vi "Fetch PRACH EVM Vs Subcarrier Trace Results.vi"(8 "error in (no error)":errorcluster, 9 "Result Type (Current)":i32(ring) items=["Current"=0, "Average"=1, "Maximum"=4], 10 "Instance (1)":T1=1, 11 "VISA resource name":refnum<visa-resource-name>) -> (0 "error out":errorcluster, 1 "Results":dbl[](array[numeric]) format="%^.3e", 2 "Reliability":i32, 3 "VISA resource name out":refnum<visa-resource-name>)   [LabVIEW 2020, in "Rohde&Schwarz CMWXP NR FR1 Measurement.lvlib"]
doc: "Returns the values of the EVM vs subcarrier traces. Each value is averaged over the samples in one preamble subcarrier.\n\nAttributes:\nRSCMWXPNRFR1M_ATTR_FETCH_PRACH_EVM_VS_SUBCARRIER_CURRENT_TRACE_RESULTS\nRSCMWXPNRFR1M_ATTR_FETCH_PRACH_EVM_VS_SUBCARRIER_AVERAGE_TRACE_RESULTS\nRSCMWXPNRFR1M_ATTR_FETCH_PRACH_EVM_VS_SUBCARRIER_MAXIMUM_TRACE_RESULTS\n\nRemote-control commands:\nFETCh:NRSub:MEAS<i>:PRACh:TRACe:EVM:CURRent?\nFETCh:NRSub:MEAS<i>:PRACh:TRACe:EVM:AVERage?\nFETCh:NRSub:MEAS<i>:PRACh:TRACe:EVM:MAXimum?"
uses:
  <instrlib>/Rohde&Schwarz CMWXP NR FR1 Measurement/Rohde&Schwarz CMWXP NR FR1 Measurement.lvlib
  <instrlib>/Rohde&Schwarz CMWXP NR FR1 Measurement/Private/_Instance.ctl
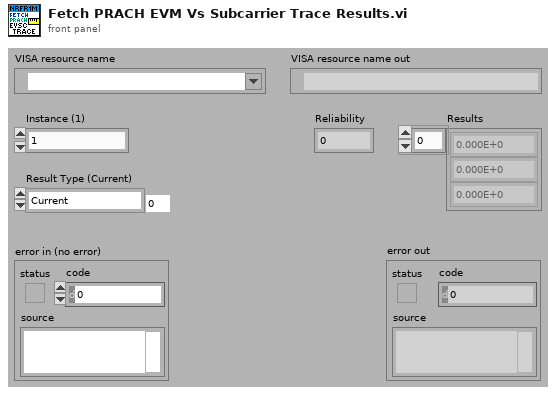
[diagram p1: front panel]
types:
  T1 = typedef "Rohde&Schwarz CMWXP NR FR1 Measurement.lvlib/_Instance.ctl" = i32
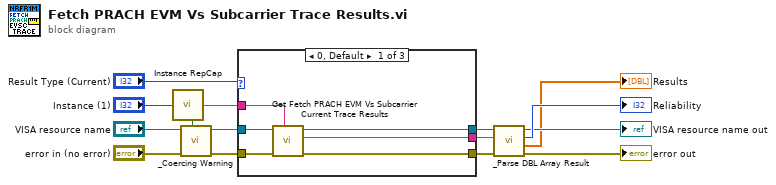
[diagram p0: block diagram]
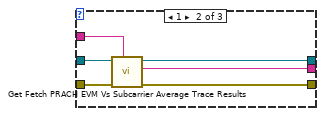
[diagram p2: hidden frame]
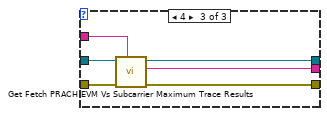
[diagram p3: hidden frame]
diagram:
  n1 = call <instrlib>:"Instance RepCap.vi"("Instance In"="Instance (1)") -> ("In Range?"=w15:bool, "RepCap Identifier Out"=w12:string)  [unwired: 1 in]
  n2 = call <instrlib>:"_Coercing Warning.vi"("In Range?"=w15, "error in (no error)"="error in (no error)", "VISA resource name"="VISA resource name") -> ("error out"=w13:errorcluster, "VISA resource name out"=w14:refnum<visa-resource-name>)  [unwired: 7 in]
  n3 = case shown="0, Default" "Result Type (Current)" {
    tunnel: w14 -> [w21 w27 w32]
    tunnel: w13 -> [w20 w26 w33]
    tunnel: w12 -> [w19 w25 w28]
    tunnel: [w18 w22 w29] -> w11
    tunnel: [w17 w24 w31] -> w9
    tunnel: [w16 w23 w30] -> w10
    frame 0, Default {
      n4 = call "Get Fetch PRACH EVM Vs Subcarrier Current Trace Results"("Repeated Capabilities"=w19, "error in (no error)"=w20, "instrument handle"=w21) -> ("error out"=w18:errorcluster, "Fetch PRACH EVM Vs Subcarrier Current Trace Results"=w16:string, "instrument handle out"=w17:refnum<visa-resource-name>)  [unwired: 6 in]
    }
    frame 1 {
      n5 = call "Get Fetch PRACH EVM Vs Subcarrier Average Trace Results"("Repeated Capabilities"=w25, "error in (no error)"=w26, "instrument handle"=w27) -> ("error out"=w22:errorcluster, "Fetch PRACH EVM Vs Subcarrier Average Trace Results"=w23:string, "instrument handle out"=w24:refnum<visa-resource-name>)  [unwired: 6 in]
    }
    frame 4 {
      n6 = call "Get Fetch PRACH EVM Vs Subcarrier Maximum Trace Results"("Repeated Capabilities"=w28, "error in (no error)"=w33, "instrument handle"=w32) -> ("error out"=w29:errorcluster, "Fetch PRACH EVM Vs Subcarrier Maximum Trace Results"=w30:string, "instrument handle out"=w31:refnum<visa-resource-name>)  [unwired: 6 in]
    }
  }
  n7 = call <instrlib>:"_Parse DBL Array Result.vi"("error in (no error)"=w11, "Input String"=w10, "VISA resource name"=w9) -> ("error out"=→"error out":errorcluster, "Results"=→"Results":dbl[], "Reliability"=→"Reliability":i32, "VISA resource name out"=→"VISA resource name out":refnum<visa-resource-name>)  [unwired: 5 in]
